vi "RT sender&receiver.vi"() -> ()   [LabVIEW 2017]
panel:
  out "Number Received from Host":i32
  in  "stop":bool
  out "Sent String to Host":string
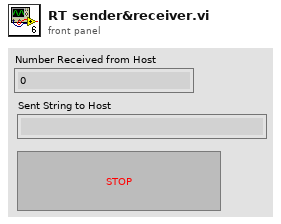
[diagram p1: front panel]
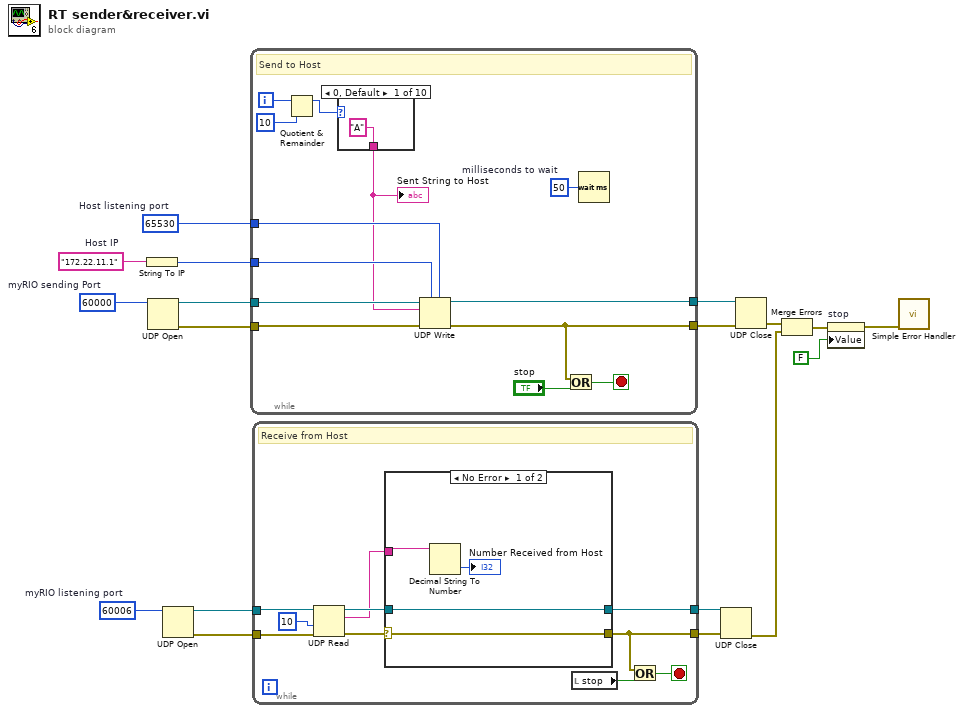
[diagram p0: block diagram]
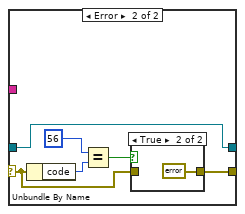
[diagram p2: hidden frame]
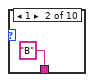
[diagram p4: hidden frame]
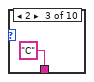
[diagram p5: hidden frame]
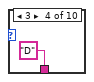
[diagram p6: hidden frame]
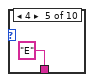
[diagram p7: hidden frame]
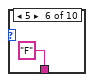
[diagram p8: hidden frame]
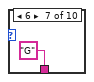
[diagram p9: hidden frame]
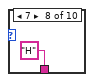
[diagram p10: hidden frame]
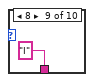
[diagram p11: hidden frame]
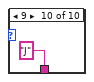
[diagram p12: hidden frame]
diagram:
  w8 = u16 60006  # myRIO listening port
  w13 = u16 65530  # Host listening port
  w15 = "172.22.11.1"  # Host IP
  w18 = u16 60000  # myRIO sending Port
  n1 = String To IP(1:w15) -> (0:w14:u32)
  n2 = UDP Open(11:w18) -> (port=w16:refnum<k16>, 0:w17:errorcluster)  [unwired: 4 in, 1 out]
  n3 = UDP Open(11:w8) -> (port=w10:refnum<k16>, 0:w9:errorcluster)  [unwired: 4 in, 1 out]
  n4 = while {
    tunnel: w17 -> [w29]
    tunnel: w16 -> [w30]
    tunnel: w14 -> [w28]
    tunnel: w13 -> [w27]
    tunnel: [w26] -> w12
    tunnel: [w24] -> w11
    i -> [w22]
    stop <- w25 stop-if-true
    w31 = u32 50  # milliseconds to wait
    # "Send to Host"
    n5 = Quotient & Remainder(x=w22, y=10) -> (x-y*floor(x/y)=w20:i32)  [unwired: 1 out]
    n6 = case shown="0, Default" w20 {
      tunnel: ["A" "B" "C" "D" "E" "F" "G" "H" "I" "J"] -> w19
      frame 0, Default {
      }
      frame 1 {
      }
      frame 2 {
      }
      frame 3 {
      }
      frame 4 {
      }
      frame 5 {
      }
      frame 6 {
      }
      frame 7 {
      }
      frame 8 {
      }
      frame 9 {
      }
    }
    "Sent String to Host" <- w19
    n7 = UDP Write(address=w28, port or service name=w27, connection ID=w30, data in=w19, 8:w29) -> (error out=w24:errorcluster, 3:w26:refnum<k16>)  [unwired: 1 in]
    n8 = Or(x=w24, y="stop") -> (x .or. y?=w25:bool)
    n9 = Wait (ms)(milliseconds to wait=w31) -> ()  [unwired: 1 out]
  }
  n10 = while {
    tunnel: w10 -> [w51]
    tunnel: w9 -> [w50]
    tunnel: [w43] -> w7
    tunnel: [w45] -> w6
    stop <- w44 stop-if-true
    # "Receive from Host"
    n11 = UDP Read(connection ID=w51, timeout ms (25000)=10, 8:w50) -> (data out=w46:string, error out=w48:errorcluster, 3:w47:refnum<k16>)  [unwired: 1 in, 2 out]
    n12 = case shown="No Error" w48 {
      selector: w48 -> [w55 w57]
      tunnel: w47 -> [w54 w56]
      tunnel: w46 -> [w53 _]
      tunnel: [w55 w58] -> w43
      tunnel: [w54 w56] -> w45
      frame No Error {
        n13 = Decimal String To Number(string=w53) -> (number=→"Number Received from Host":i32)  [unwired: 2 in, 1 out]
      }
      frame Error {
        n14 = Unbundle By Name(w57) -> ("code"=w61:i32)
        n15 = Equal?(x=56, y=w61) -> (x = y?=w59:bool)
        n16 = case shown="True" w59 {
          tunnel: [w62 errorcluster {"status"=FALSE, "code"=0, "source"=""} ("error constant")] -> w58
          tunnel: w57 -> [w62 _]
          frame False {
          }
          frame True {
          }
        }
      }
    }
    n17 = local read "stop"() -> (w42:bool)
    n18 = Or(x=w43, y=w42) -> (x .or. y?=w44:bool)
  }
  n19 = UDP Close(connection ID=w6, 8:w7) -> (error out=w2:errorcluster)  [unwired: 1 out]
  n20 = UDP Close(connection ID=w12, 8:w11) -> (error out=w5:errorcluster)  [unwired: 1 out]
  n21 = Merge Errors(w5, w2) -> (w4:errorcluster)
  n22 = property on="stop" class="Bool (strict)"(error in=w4, "Value"=FALSE ("stop")) -> (error out=w3:errorcluster)  [unwired: 1 in, 1 out]
  n23 = call <vilib>:"Simple Error Handler.vi"("error in (no error)"=w3) -> ()  [unwired: 4 in, 5 out]
